vi "Retain Wire Values.vi"(8 "error in":errorcluster, 9 "Retain Wire Values":bool, 10 "Selected VIs":string[](array[string]), 11 "Application in":refnum<vi>) -> (0 "error out":errorcluster)   [LabVIEW 2013, in "LVTM.lvlib"]
uses:
  LVTM.lvlib
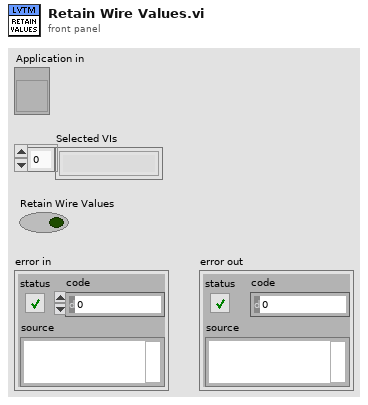
[diagram p1: front panel]
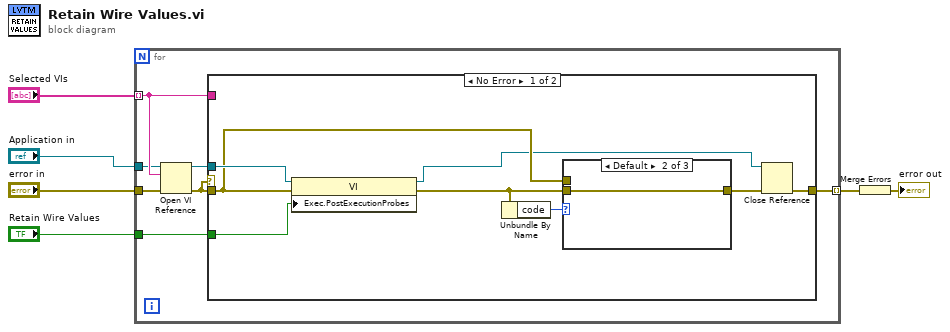
[diagram p0: block diagram]
diagram:
  n1 = for {
    tunnel: "Selected VIs" -> [w10] mode=indexing
    tunnel: "error in" -> [w12]
    tunnel: [w11] -> w1 mode=indexing
    tunnel: "Application in" -> [w9]
    tunnel: "Retain Wire Values" -> [w8]
    n2 = Open VI Reference(application reference (local)=w9, vi path=w10, error in (no error)=w12) -> (vi reference=w13:refnum<vi>, error out=w7:errorcluster)  [unwired: 3 out]
    n3 = case shown="No Error" w7 {
      tunnel: w13 -> [w21 _]
      tunnel: [w20 _] -> w11
      tunnel: w10 -> [_ _]
      tunnel: w7 -> [w16 _]
      tunnel: w8 -> [w14 _]
      frame No Error {
        n4 = property class="VI"(reference=w21, error in=w16, "Exec.PostExecutionProbes"=w14) -> (reference out=w15:refnum<vi>, error out=w17:errorcluster)
        n5 = Unbundle By Name(w17) -> ("code"=w19:i32)
        n6 = case shown="Default" w19 {
          tunnel: [w22 w23 w24] -> w18
          tunnel: w17 -> [w22 w23 _]
          tunnel: w16 -> [_ _ w24]
          frame 0 {
          }
          frame Default {
          }
          frame 1035 {
            # "Operation is invalid for this type of VI.\nIgnore Error."
          }
        }
        n7 = Close Reference(reference=w15, error in (no error)=w18) -> (error out=w20:errorcluster)
      }
      frame Error {
        # "This VI is no longer in the memory"
      }
    }
  }
  n8 = Merge Errors(w1) -> (→"error out":errorcluster)
